vi "Channel Select.vi"(6 "Path In":path, 8 "error in (no error)":errorcluster, 9 "Previous Selection":string[](array[string])=["Populating List..."], 10 "Messaage":string, 11 "Gateway IP Address":string) -> (0 "error out":errorcluster, 2 "Path to System Definition File":path, 3 "Channel Paths":string[](array[string]))   [LabVIEW 2014]
doc: "Opens a reference to a VeriStand Workspace and populates the list with availables channels. The user can select and channel and then click OK."
uses:
  <vilib>/NI Veristand/Execution/Workspace/NI_VS Workspace ExecutionAPI.lvlib
  <userlib>/Simple SysDef/Simple SysDef API.lvlib
panel:
  in  "error in (no error) 2":errorcluster
  in  "Cancel":bool
  in  "Select":bool
  in  "VeriStand Channels":i32[](listbox)
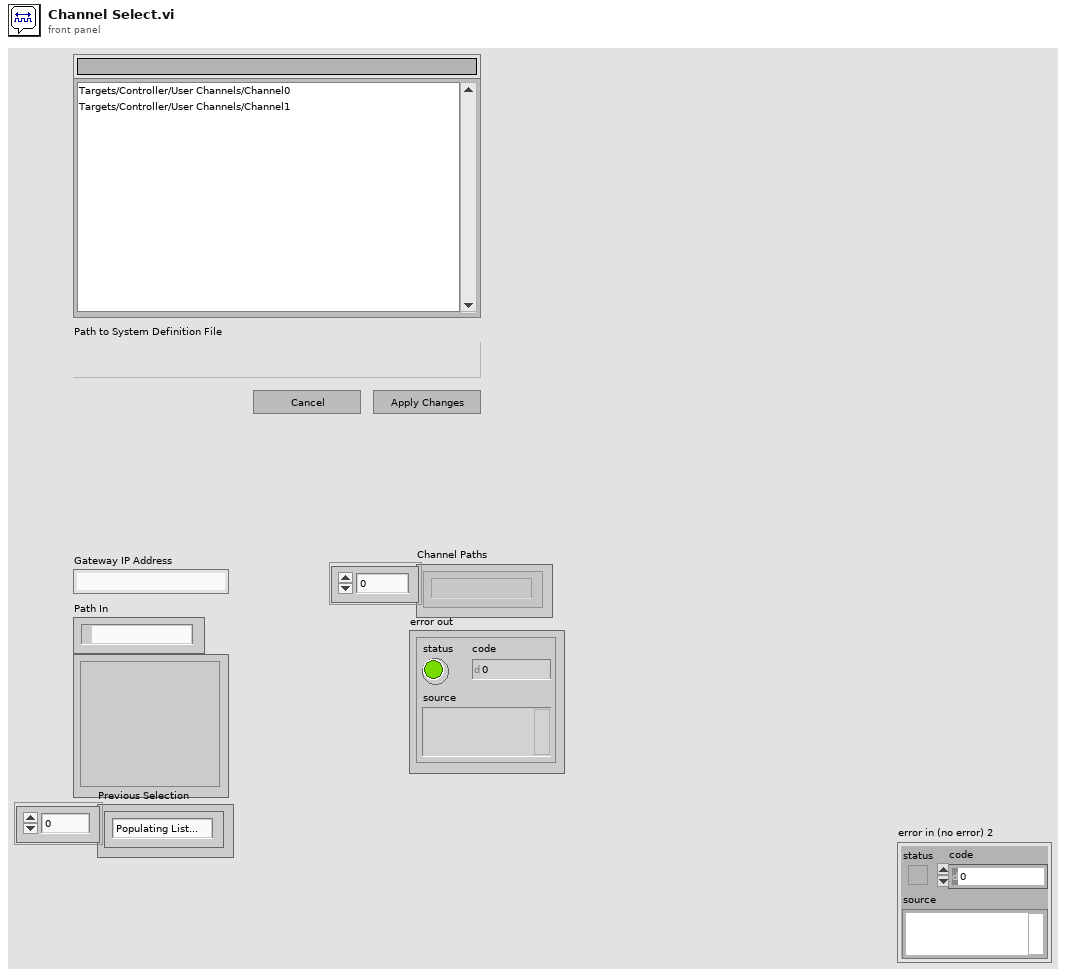
[diagram p1: front panel]
types:
  T1 = typedef "NI_VS Workspace ExecutionAPI.lvlib/WorkspaceAPI.ctl" = refnum<k24>
  T2 = typedef "NI_VS Workspace ExecutionAPI.lvlib/NodeInfo.ctl" = cluster{"Name":string, "FullPath":string, "Type":string, "IsChannel":bool, "Channel":cluster{"Unit":string, "Readable":bool, "Writable":bool, "Faultable":bool, "Scalable":bool, "RowDim":u32, "ColumnDim":u32}, "IsWaveform":bool, "Waveform":cluster{"DataType":T3}}
  T3 = typedef "NI_VS Workspace ExecutionAPI.lvlib/Waveform Data Type.ctl" = enum16{"Double", "ComplexDouble"}
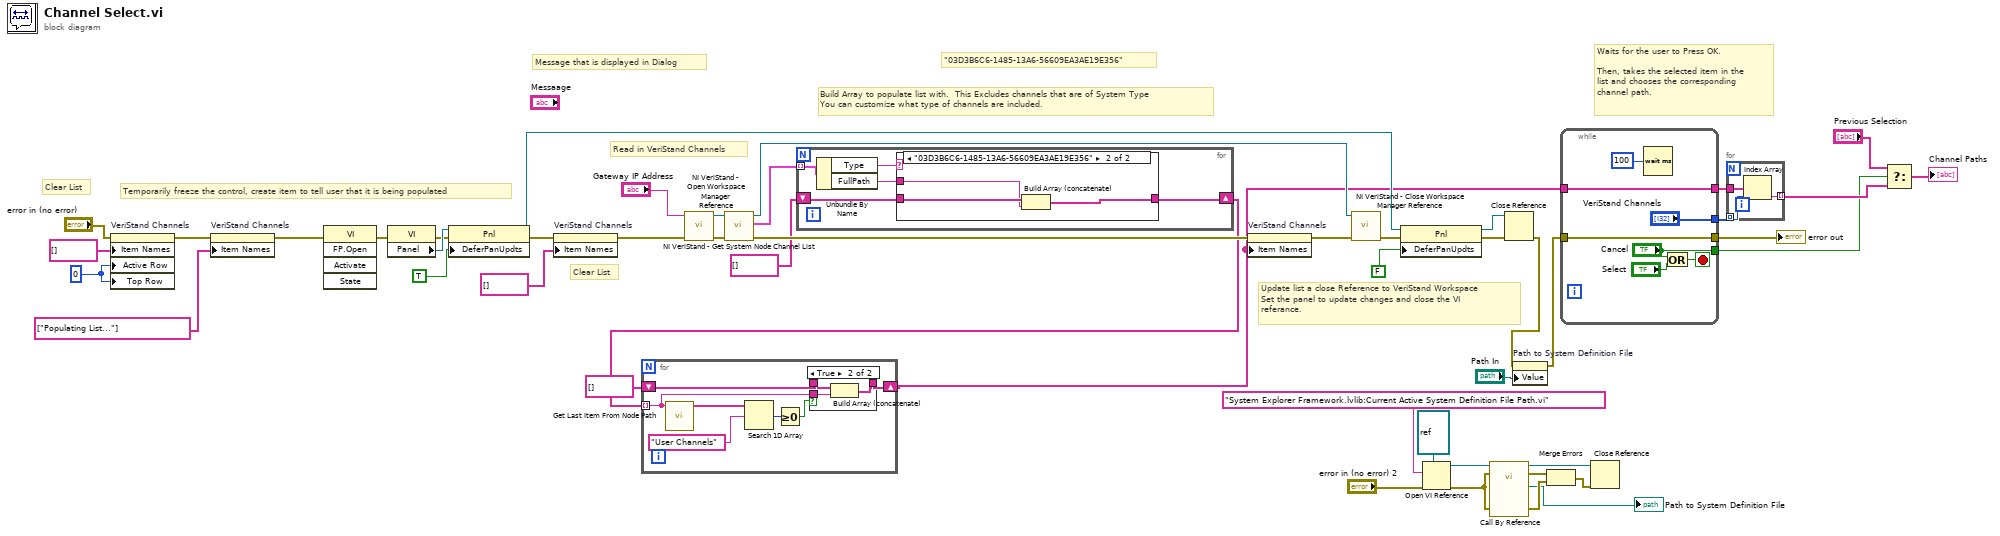
[diagram p0: block diagram]
diagram:
  w25 = 0 ("Active Row:Active Row Number")
  # "\"03D3B6C6-1485-13A6-56609EA3AE19E356\""
  # "Message that is displayed in Dialog"
  # "Waits for the user to Press OK.\n\nThen, takes the selected item in the \nlist and chooses the corresponding\nchannel path."
  # "Update list a close Reference to VeriStand Workspace\nSet the panel to update changes and close the VI \nreferance."
  # "Clear List"
  # "Build Array to populate list with.  This Excludes channels that are of System Type\nYou can customize what type of channels are included."
  # "Read in VeriStand Channels"
  # "Clear List"
  # "Temporarily freeze the control, create item to tell user that it is being populated"
  n1 = property on="VeriStand Channels" class="LstBox (strict)"(error in="error in (no error)", "Item Names"=string[] [], "Active Row"=w25, "Top Row"=w25) -> (error out=w39:errorcluster)  [unwired: 1 in, 1 out]
  n2 = property on="VeriStand Channels" class="LstBox (strict)"(error in=w39, "Item Names"=string[] ["Populating List..."]) -> (error out=w37:errorcluster)  [unwired: 1 in, 1 out]
  n3 = invoke class="VI" method="FP.Open"(error in=w37) -> (error out=w49:errorcluster)  [unwired: 4 in, 4 out]
  n4 = property class="VI"(error in=w49) -> (error out=w47:errorcluster, "Panel"=w48:refnum<vi>)  [unwired: 1 in, 1 out]
  n5 = property class="Pnl"(reference=w48, error in=w47, "DeferPanUpdts"=TRUE ("Defer Panel Updates")) -> (reference out=w42:refnum<vi>, error out=w35:errorcluster)
  n6 = property on="VeriStand Channels" class="LstBox (strict)"(error in=w35, "Item Names"=string[] []) -> (error out=w22:errorcluster)  [unwired: 1 in, 1 out]
  n7 = call <vilib>:"NI VeriStand - Open Workspace Manager Reference.vi"("error in (no error)"=w22, "Gateway IP Address (\"\": localhost)"="Gateway IP Address") -> ("error out"=w24:errorcluster, "WorkspaceManager"=w23:T1)  [unwired: 8 in]
  n8 = call <vilib>:"NI VeriStand - Get System Node Channel List.vi"("error in (no error)"=w24, "WorkspaceManager in"=w23) -> ("error out"=w34:errorcluster, "Channels"=w41:T2[], "WorkspaceManager out"=w32:T1)  [unwired: 7 in]
  n9 = for {
    tunnel: w41 -> [w54] mode=indexing
    shift-right: [w51] -> w13
    shift-left: string[] [] -> [w52]
    n10 = Unbundle By Name(w54) -> ("Type"=w53:string, "FullPath"=w50:string)
    n11 = case shown="\"03D3B6C6-1485-13A6-56609EA3AE19E356\"" w53 {
      tunnel: w52 -> [w55 w58]
      tunnel: [w55 w57] -> w51
      tunnel: w50 -> [_ w56]
      frame "", Default {
      }
      frame "03D3B6C6-1485-13A6-56609EA3AE19E356" {
        n12 = Build Array (concatenate)(w58, w56) -> (w57:string[])
      }
    }
  }
  n13 = for {
    tunnel: w13 -> [w60] mode=indexing
    shift-right: [w62] -> w11
    shift-left: string[] [] -> [w61]
    n14 = call <userlib>:"Get Last Item From Node Path.vi"("Name"=w60) -> ("First Items"=w65:string[])  [unwired: 9 in, 1 out]
    n15 = Search 1D Array(1D array=w65, element="User Channels") -> (index of element=w63:i32)  [unwired: 1 in]
    n16 = Greater Or Equal To 0?(x=w63) -> (x >= 0?=w59:bool)
    n17 = case shown="True" w59 {
      tunnel: [w66 w69] -> w62
      tunnel: w61 -> [w66 w68]
      tunnel: w60 -> [_ w67]
      frame False {
      }
      frame True {
        n18 = Build Array (concatenate)(w68, w67) -> (w69:string[])
      }
    }
  }
  n19 = property on="VeriStand Channels" class="LstBox (strict)"(error in=w34, "Item Names"=w11) -> (error out=w33:errorcluster)  [unwired: 1 in, 1 out]
  n20 = call <vilib>:"NI VeriStand - Close Workspace Manager Reference.vi"("error in (no error)"=w33, "WorkspaceManager"=w32) -> ("error out"=w31:errorcluster)  [unwired: 9 in]
  n21 = property class="Pnl"(reference=w42, error in=w31, "DeferPanUpdts"=FALSE ("Defer Panel Updates")) -> (reference out=w45:refnum<vi>, error out=w44:errorcluster)
  n22 = Open VI Reference(type specifier VI Refnum (for type only)=refnum<vi> refnum, vi path="System Explorer Framework.lvlib:Current Active System Definition File Path.vi", error in (no error)="error in (no error) 2") -> (vi reference=w4:refnum<vi>, error out=w6:errorcluster)  [unwired: 3 in]
  n23 = call-by-ref "?"(reference=w4, error in=w6, 8:"error in (no error)"=w6) -> (reference out=w10:refnum<vi>, error out=w7:errorcluster, 0:"error out"=w8:errorcluster, "Active System Definition Path"=→"Path to System Definition File":path)  [unwired: 9 in]
  n24 = Close Reference(reference=w45, error in (no error)=w44) -> (error out=w15:errorcluster)
  n25 = property on="Path to System Definition File" class="Path"(error in=w15, "Value"="Path In") -> (error out=w14:errorcluster)  [unwired: 1 in, 1 out]
  n26 = Merge Errors(w7, w8) -> (w9:errorcluster)
  n27 = while {
    tunnel: w14 -> [w73]
    tunnel: w11 -> [w74]
    tunnel: ["VeriStand Channels"] -> w28
    tunnel: [w74] -> w29
    tunnel: [w73] -> w26
    tunnel: ["Cancel"] -> w17
    stop <- w71 stop-if-true
    n28 = Wait (ms)(milliseconds to wait=u32 100) -> ()  [unwired: 1 out]
    n29 = Or(x="Cancel", y="Select") -> (x .or. y?=w71:bool)
  }
  "error out" <- w26
  n30 = Close Reference(reference=w10, error in (no error)=w9) -> ()  [unwired: 1 out]
  n31 = for {
    tunnel: w29 -> [w79]
    tunnel: w28 -> [w78] mode=indexing
    tunnel: [w77] -> w19 mode=indexing
    n32 = Index Array(array=w79, index=w78) -> (element=w77:string)
  }
  n33 = Select(t="Previous Selection", s=w17, f=w19) -> (s? t:f=→"Channel Paths":string[])
